vi "FSN_Query.vi"(0 "System no.":i32=1 min=1 step=1, 2 "Queried axes":string[](array[string])=["x", "y", "z", "u", "v", "w"], 5 "error in":errorcluster) -> (15 "Maximum level":dbl=1.0 format="%.3f", 16 "Position values":dbl[](array[numeric]) format="%.6f", 19 "error out":errorcluster)   [LabVIEW 2020]
doc: "Returns the maximum level found during the last FSN scan and the coordinates where it was found. \n\nC-887, F-206, M-8X0: Only for GCS syntax version = GCS 1.0 (check with CSV?.vi. If CSV?.vi is not supported, syntax version is GCS 1.0)."
panel:
  # "Returns the maximum level found during the last FSN scan \nand the coordinates where it was found."
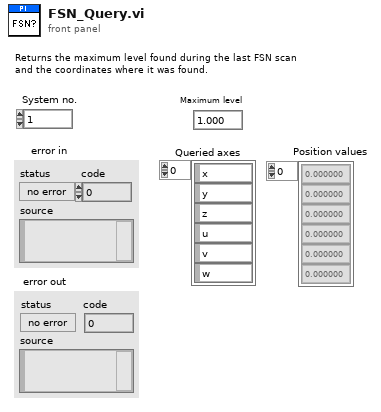
[diagram p1: front panel]
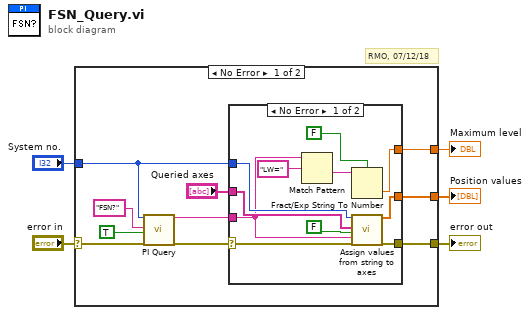
[diagram p0: block diagram]
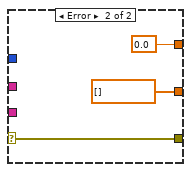
[diagram p2: hidden frame]
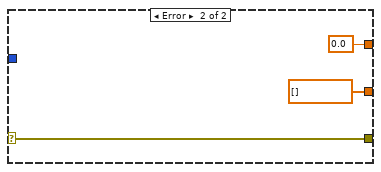
[diagram p3: hidden frame]
diagram:
  # "RMO, 07/12/18"
  n1 = case shown="No Error" "error in" {
    selector: "error in" -> [w7 w30]
    tunnel: "System no." -> [w13 _]
    tunnel: [w11 w30] -> w4
    tunnel: [w10 0.0] -> w3
    tunnel: [w9 dbl[] [] ("Values")] -> w2
    frame No Error {
      n2 = call "PI Query.vi"("System no."=w13, "String to send"="FSN?", "Attach termination char.?"=TRUE ("Attach Linefeed?"), "error in"=w7) -> ("String read"=w8:string, "error out"=w6:errorcluster)  [unwired: 3 in, 11 out]
      n3 = case shown="No Error" w6 {
        selector: w6 -> [w16 w27]
        tunnel: [w23 0.0] -> w10
        tunnel: w8 -> [w19 _]
        tunnel: w13 -> [w22 _]
        tunnel: "Queried axes" -> [w21 _]
        tunnel: [w18 w27] -> w11
        tunnel: [w17 dbl[] [] ("Values")] -> w9
        frame No Error {
          n4 = Match Pattern(string=w19, regular expression="LW=") -> (after substring=w25:string)  [unwired: 4 out]
          n5 = Fract/Exp String To Number(use system decimal point (T)=FALSE, string=w25) -> (number=w23:dbl)  [unwired: 3 out]
          n6 = call "Assign values from string to axes.vi"("System no."=w22, "Queried axes"=w21, "All axes queried?"=FALSE, "Input String"=w19, "error in"=w16) -> ("Values"=w17:dbl[], "error out"=w18:errorcluster)  [unwired: 1 in, 12 out]
        }
        frame Error {
        }
      }
    }
    frame Error {
    }
  }
  "error out" <- w4
  "Maximum level" <- w3
  "Position values" <- w2
